vi "OCV Close Camera.vi"(8 "error in (no error)":errorcluster) -> (0 "error out":errorcluster)   [LabVIEW 2018, in "OpenCVcamLV.lvlib"]
uses:
  OpenCVcamLV.lvlib
  LVopenCVcamDLL.dll
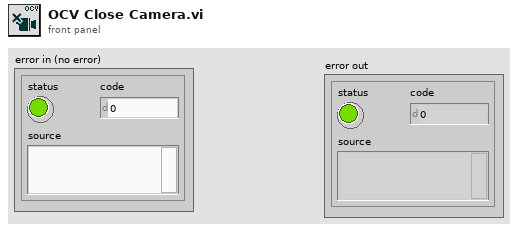
[diagram p1: front panel]
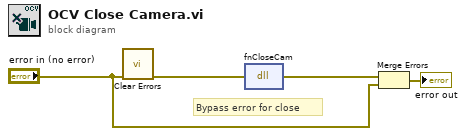
[diagram p0: block diagram]
diagram:
  # "Bypass error for close"
  n1 = call <vilib>:"Clear Errors.vi"("error in (no error)"="error in (no error)") -> ("error out"=w1:errorcluster)  [unwired: 5 in, 1 out]
  n2 = dll-call lib="C:/Users/Andrey/Desktop/OpenCVcamLV/LVopenCVcamDLL.dll" fn="fnCloseCam"(error in=w1) -> (error out=w4:errorcluster)  [unwired: 3 in, 1 out]
  n3 = Merge Errors(w4, "error in (no error)") -> (→"error out":errorcluster)
